vi "Test.vi"   [LabVIEW 2015]
doc: "This VI is called when test mode begins, and will automatically be terminated when it ends. You can add manual or automatic tests and invoke them from the dashboard."
uses:
  <vilib>/Rock Robotics/WPI/Relay/WPI_RelayValue.ctl
  Robot Global Data.vi
  <vilib>/Rock Robotics/WPI/Utilities/WPI_GetSetVariantRefNum.vi
types:
  T1 = typedef "WPI_RelayValue.ctl" = enum16{"Off", "On", "Forward", "Reverse"}
  T2 = typedef "WPI_RelayDevRef.ctl" = cluster{"DevStatus":errorcluster, "Relay Channel":T3, "Relay Direction":T4}
  T3 = typedef "FPGA_DIORelayChannel.ctl" = enum8{"Relay 0", "Relay 1", "Relay 2", "Relay 3", "Invalid"}
  T4 = typedef "WPI_RelayDirection.ctl" = enum16{"Both directions", "Forward only", "Reverse only"}
  T5 = typedef "WPI_CompressorDevRef.ctl" = cluster{"DevStatus":errorcluster, "Pneumatics Control Module":u8}
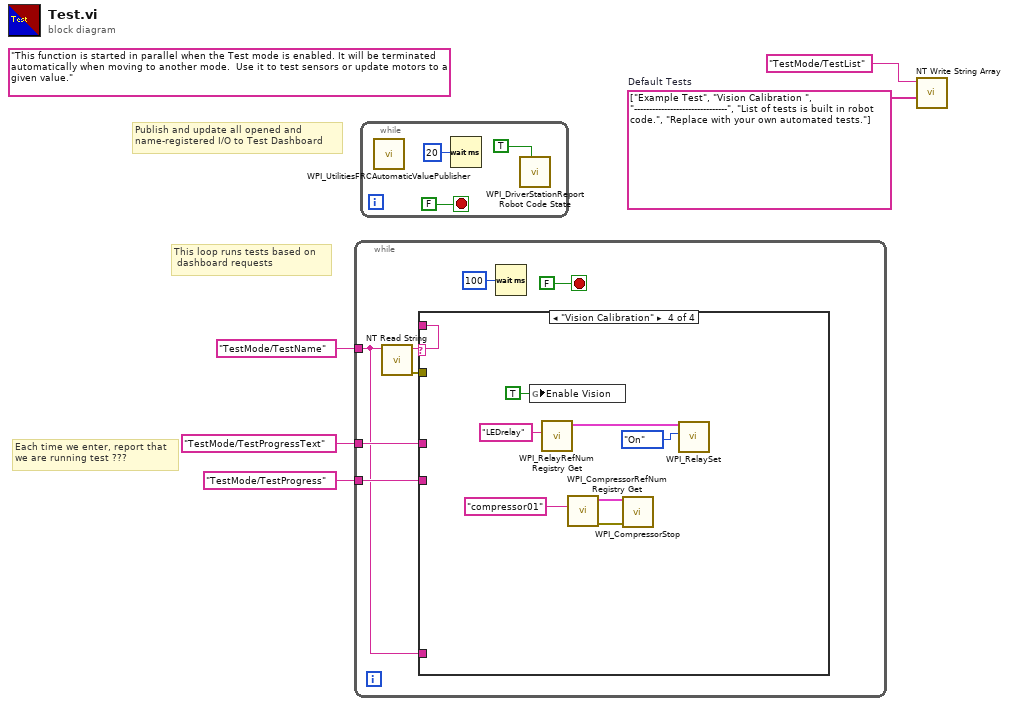
[diagram p0: block diagram]
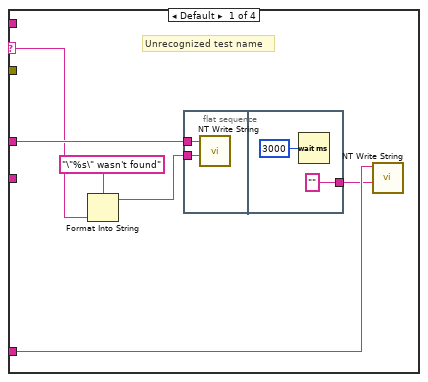
[diagram p2: hidden frame]
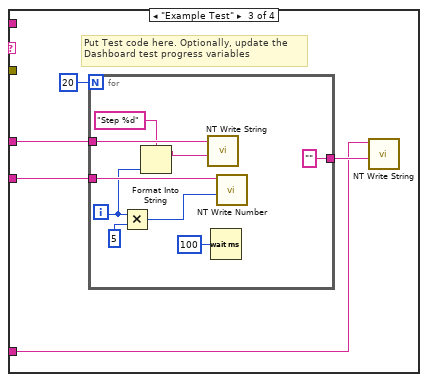
[diagram p4: hidden frame]
diagram:
  w2 = string[] ["Example Test", "Vision Calibration ", "-------------------------------", "List of tests is built in robot code.", "Replace with your own automated tests."]  # Default Tests
  (unwired) "This function is started in parallel when the Test mode is enabled. It will be terminated automatically when moving to another mode.  Use it to test sensors or update motors to a given value."
  # "This loop runs tests based on \n dashboard requests"
  # "Publish and update all opened and\nname-registered I/O to Test Dashboard"
  # "Each time we enter, report that\nwe are running test ???"
  n1 = while {
    tunnel: "TestMode/TestName" ("Name") -> [w7]
    tunnel: "TestMode/TestProgressText" ("Name") -> [w10]
    tunnel: "TestMode/TestProgress" ("Name") -> [w9]
    stop <- FALSE stop-if-true
    n2 = call <vilib>:"NT Read String.vi"("Name"=w7) -> ("error out"=w6:errorcluster, "String"=w8:string)  [unwired: 9 in]
    n3 = case shown="\"Vision Calibration\"" w8 {
      selector: w8 -> [w17 _ _ _]
      tunnel: w7 -> [w14 _ w23 _]
      tunnel: w10 -> [w18 _ w26 _]
      tunnel: w9 -> [_ _ w27 _]
      tunnel: w8 -> [_ _ _ _]
      tunnel: w6 -> [_ _ _ _]
      frame Default {
        # "Unrecognized test name"
        n4 = Format Into String(format string="\"%s\" wasn't found" ("Name"), w17) -> (resulting string=w16:string)  [unwired: 2 in, 1 out]
        n5 = flat-sequence {
          tunnel: w18 -> [w19]
          tunnel: w16 -> [w20]
          tunnel: ["" ("Name")] -> w13
          frame #0 {
            n6 = call <vilib>:"NT Write String.vi"("String"=w20, "Name"=w19) -> ()  [unwired: 9 in, 1 out]
          }
          frame #1 {
            n7 = Wait (ms)(milliseconds to wait=u32 3000) -> ()  [unwired: 1 out]
          }
        }
        n8 = call <vilib>:"NT Write String.vi"("String"=w13, "Name"=w14) -> ()  [unwired: 9 in, 1 out]
      }
      frame "" {
        # "No test to run"
      }
      frame "Example Test" {
        # "Put Test code here. Optionally, update the\nDashboard test progress variables"
        n9 = for {
          N: 20 -> [_]
          tunnel: w27 -> [w36]
          tunnel: w26 -> [w34]
          tunnel: ["" ("String")] -> w24
          i -> [w31]
          n10 = Multiply(x=w31, y=u32 5 ("milliseconds to wait")) -> (x*y=w32:u32)
          n11 = Format Into String(format string="Step %d", w31) -> (resulting string=w29:string)  [unwired: 2 in, 1 out]
          n12 = call <vilib>:"NT Write String.vi"("String"=w29, "Name"=w34) -> ()  [unwired: 9 in, 1 out]
          n13 = Wait (ms)(milliseconds to wait=u32 100) -> ()  [unwired: 1 out]
          n14 = call <vilib>:"NT Write Number.vi"("Numeric"=w32, "Name"=w36) -> ()  [unwired: 9 in, 1 out]
        }
        n15 = call <vilib>:"NT Write String.vi"("String"=w24, "Name"=w23) -> ()  [unwired: 9 in, 1 out]
      }
      frame "Vision Calibration" {
        n16 = global write "Robot Global Data.vi" "Enable Vision"(TRUE ("Enable Vision")) -> ()
        n17 = call <vilib>:"WPI_RelayRefNum Registry Get.vi"("refnum name"="LEDrelay") -> ("RelayDevRef"=w40:T2)  [unwired: 9 in, 1 out]
        n18 = call <vilib>:"WPI_CompressorRefNum Registry Get.vi"("refnum name"="compressor01") -> ("error out"=w39:errorcluster, "CompressorDevRef"=w38:T5)  [unwired: 9 in]
        n19 = call <vilib>:"WPI_CompressorStop.vi"("error in (no error)"=w39, "CompressorDevRef"=w38) -> ()  [unwired: 8 in, 2 out]
        n20 = call <vilib>:"WPI_RelaySet.vi"("RelayValue"=WPI_RelayValue."On", "RelayDevRef"=w40) -> ()  [unwired: 8 in, 2 out]
      }
    }
    n21 = Wait (ms)(milliseconds to wait=u32 100) -> ()  [unwired: 1 out]
  }
  n22 = while {
    stop <- FALSE stop-if-true
    n23 = call <vilib>:"WPI_UtilitiesFRCAutomaticValuePublisher.vi"() -> ()  [unwired: 12 in]
    n24 = Wait (ms)(milliseconds to wait=u32 20) -> ()  [unwired: 1 out]
    n25 = call <vilib>:"WPI_DriverStationReport Robot Code State.vi"("Test"=TRUE ("Autonomous")) -> ()  [unwired: 10 in, 1 out]
  }
  n26 = call <vilib>:"NT Write String Array.vi"("String Array"=w2, "Name"="TestMode/TestList") -> ()  [unwired: 9 in, 1 out]
